vi "Configure Waveform (Simple).vi"(6 "DC Offset (0.00 V)":dbl, 7 "Frequency (1000 Hz)":dbl=1000.0, 8 "error in (no error)":errorcluster, 9 "Amplitude (1.0 Vpp)":dbl=1.0, 10 "Waveform Function (0: Sine)":enum16{"Sine", "Noise", "DC"}(ring), 11 "VISA resource name":refnum<visa-resource-name>) -> (0 "error out":errorcluster, 3 "VISA resource name out":refnum<visa-resource-name>)   [LabVIEW 2017, in "Keithley 3390.lvlib"]
doc: "Selects the waveform shape, frequency, amplitude, offset, and phase for a standard waveform."
uses:
  Keithley 3390.lvlib
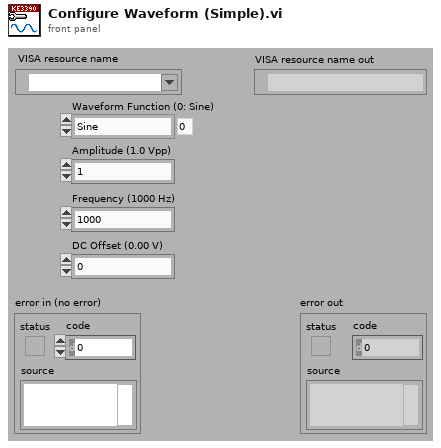
[diagram p1: front panel]
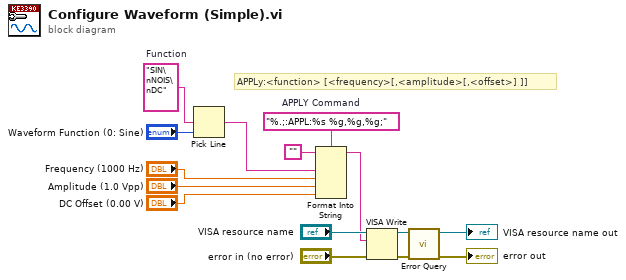
[diagram p0: block diagram]
diagram:
  w7 = "%.;:APPL:%s %g,%g,%g;"  # APPLY Command
  w8 = "SIN\nNOIS\nDC"  # Function
  # "APPLy:<function> [<frequency>[,<amplitude>[,<offset>] ]]"
  n1 = Pick Line(multi-line string=w8, line index="Waveform Function (0: Sine)") -> (output string=w6:string)  [unwired: 1 in]
  n2 = Format Into String(format string=w7, initial string="", w6, "Frequency (1000 Hz)", "Amplitude (1.0 Vpp)", "DC Offset (0.00 V)") -> (resulting string=w1:string)  [unwired: 1 in, 1 out]
  n3 = VISA Write(VISA resource name="VISA resource name", write buffer=w1, error in (no error)="error in (no error)") -> (VISA resource name out=w11:refnum<visa-resource-name>, error out=w10:errorcluster)  [unwired: 1 out]
  n4 = call "Error Query.vi"("error in (no error)"=w10, "VISA resource name"=w11) -> ("error out"=→"error out":errorcluster, "VISA resource name out"=→"VISA resource name out":refnum<visa-resource-name>)  [unwired: 6 in, 2 out]
